vi "Login.vi"(7 "Database":refnum<queue>, 8 "error in (no error)":errorcluster, 11 "System Config":T1 {"Config Settings"."Simulated Sensor Injection" scale=0.0..100.0}) -> (0 "error out":errorcluster, 3 "Simulation Mode?":bool)   [LabVIEW 2026]
uses:
  Architecture/Message Queue/Message Cluster.ctl
  controls/UI/System Config.ctl
  controls/UI/Config Settings.ctl
  controls/UI/Analog Output.ctl
  controls/UI/Units Enum.ctl
  controls/UI/Signal Enum.ctl
  controls/UI/Login Refs.ctl
  controls/UI/UI List Type.ctl
  controls/Diagnostics/Error Payload.ctl
  controls/Diagnostics/Error Cluster.ctl
  controls/Messaging Payloads/Sensor InsertRequest.ctl
  controls/Messaging Payloads/Sensor CoreData Cluster.ctl
  controls/Messaging Payloads/Operator InsertRequest.ctl
  C:/Program Files (x86)/dotnet/shared/Microsoft.NETCore.App/8.0.22/System.Security.Cryptography.dll
  Program Files (x86)/dotnet/shared/Microsoft.NETCore.App/8.0.22/System.Security.Cryptography.dll
  Architecture/Message Queue/Enqueue Message (Single).vi
  Architecture/Message Queue/Message Queue.lvlib
  Settings/Settings.lvlib
panel:
  in  "Log Out":bool
  out "Message":string
  out "Status":bool
  in  "Tab Control":enum32{"Page 1", "Sensors", "Operators"}(tab)
  in  "OK Button":bool
  in  "Cancel Button":bool
  in  "Password":string
  in  "Output Signal":T4
  in  "Units":T5
  in  "Maximum":dbl
  in  "Minimum":dbl
  in  "Serial Number":string
  in  "Model Numbers":string(combo)
  in  "Submit":bool
  in  "Submit 2":bool
  in  "New Operator Name":string
  # "ADMINISTRATOR ACCESS"
  # "Enter you administrator password to continue."
  # "Administrator access is required to manage \n           sensors and operators."
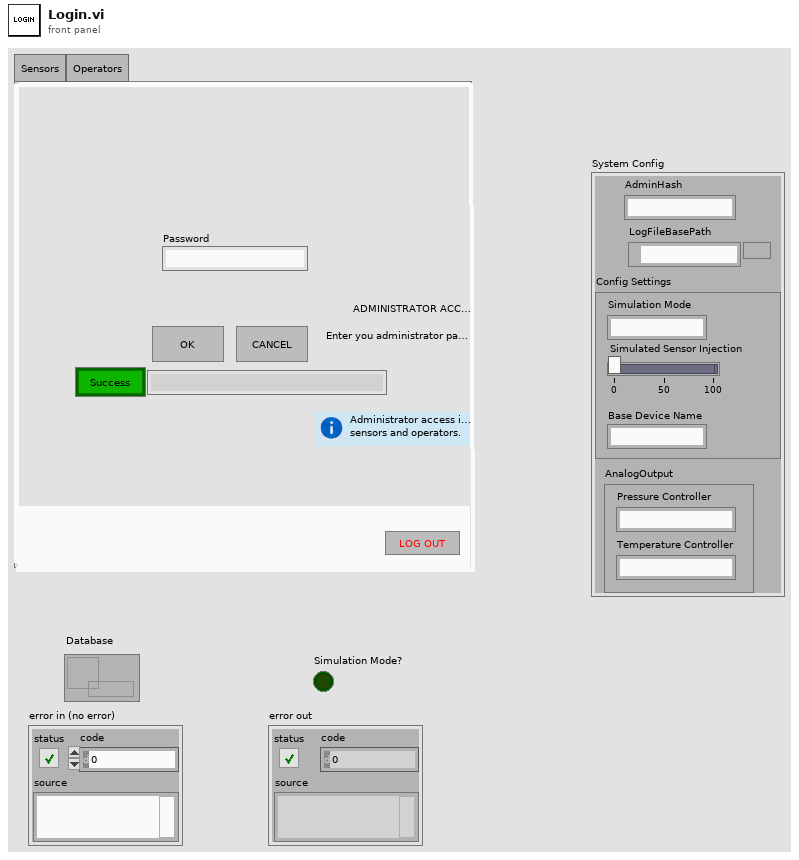
[diagram p1: front panel]
types:
  T1 = typedef "System Config.ctl" = cluster{"AdminHash":string, "LogFileBasePath ":path, "Config Settings":T2, "AnalogOutput":T3}
  T2 = typedef "Config Settings.ctl" = cluster{"Simulated Sensor Injection":dbl, "Base Device Name":string, "Simulation Mode":string}
  T3 = typedef "Settings.lvlib/Analog Output.ctl" = cluster{"Pressure Controller":string, "Temperature Controller":string}
  T4 = typedef "Signal Enum.ctl" = enum16{"4-20mA", "0-10V", "Thermocouple Type K"}
  T5 = typedef "Units Enum.ctl" = enum16{"PSI", "Deg C", "kPa", "GPM"}
  T6 = typedef "Login Refs.ctl" = cluster{"Serial Number Ref":refnum<vi>, "Submit Ref":refnum<vi>, "Clear Refnum ":refnum<vi>, "Logout Ref":refnum<vi>, "Message Ref":refnum<vi>, "Status Ref":refnum<vi>, "TabCtl Ref":refnum<vi>, "Submit Ref 2":refnum<vi>}
  T7 = enum8{"Enabled", "Disabled", "Disabled and Grayed Out"}
  T8 = typedef "UI List Type.ctl" = enum16{"Model Numbers", "Serial Numbers", "Operators", "Calibration Points", "Start Run Times"}
  T9 = typedef "Error Payload.ctl" = cluster{"Error Cluster":T10, "Message":string}
  T10 = typedef "Error Cluster.ctl" = errorcluster
  T11 = typedef "Sensor InsertRequest.ctl" = cluster{"Notifier":refnum<notifier>, "Sensor CoreData":T12}
  T12 = typedef "Settings.lvlib/Sensor CoreData Cluster.ctl" = cluster{"SensorID":i32, "SerialNumber":string, "ModelNumber":string, "Min":dbl, "Max":dbl, "Units":T5, "Output Signal":T4}
  T13 = typedef "Operator InsertRequest.ctl" = cluster{"Notifier":refnum<notifier>, "OperatorName":string, "BadgeNumber":string, "IsActive":i32}
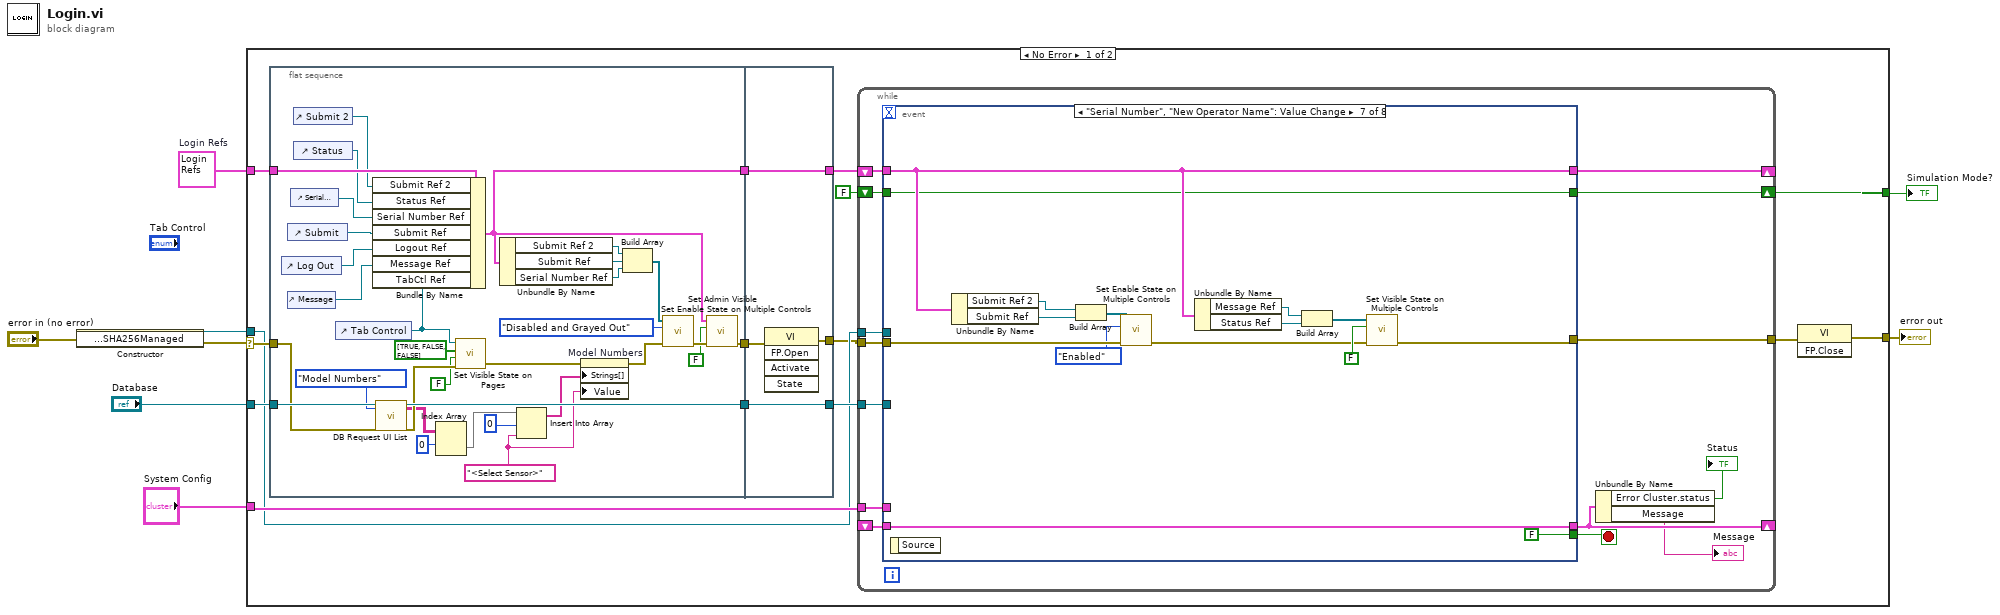
[diagram p0: block diagram]
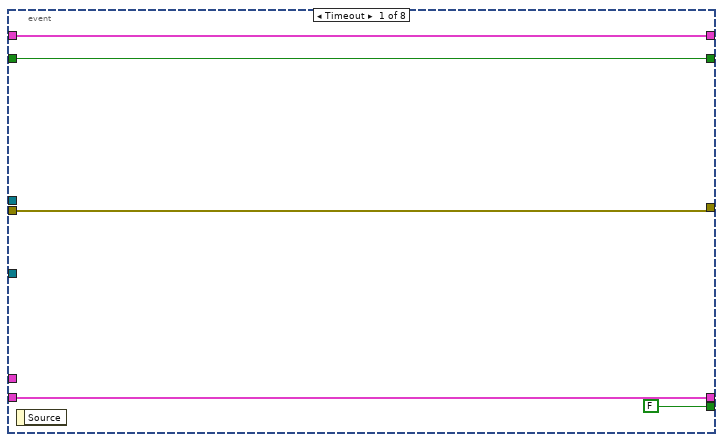
[diagram p2: hidden frame]
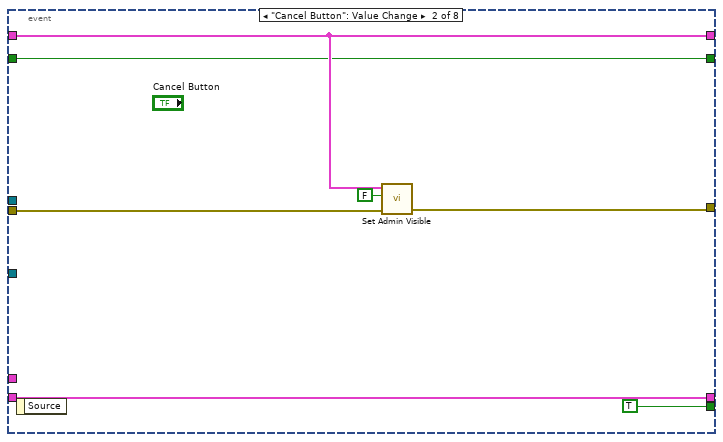
[diagram p3: hidden frame]
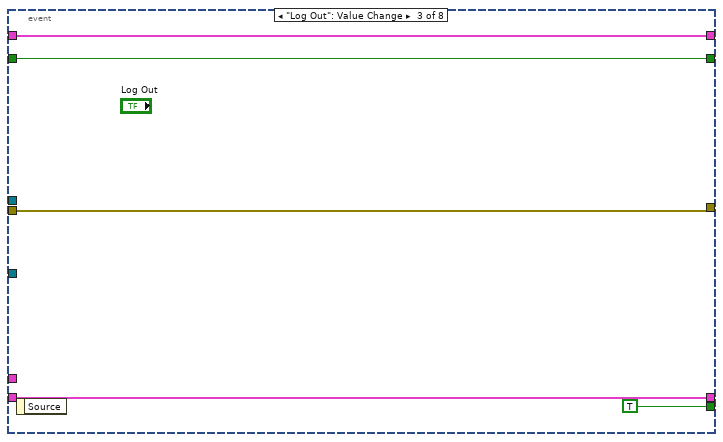
[diagram p4: hidden frame]
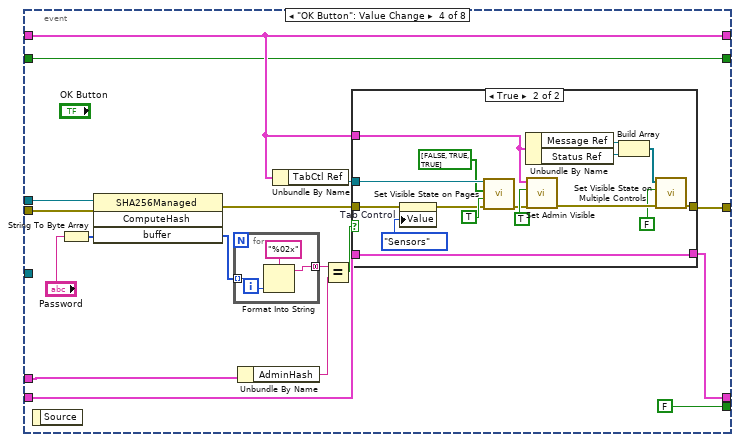
[diagram p5: hidden frame]
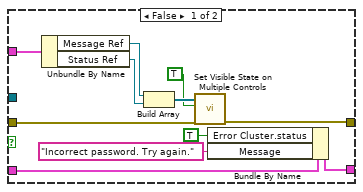
[diagram p6: hidden frame]
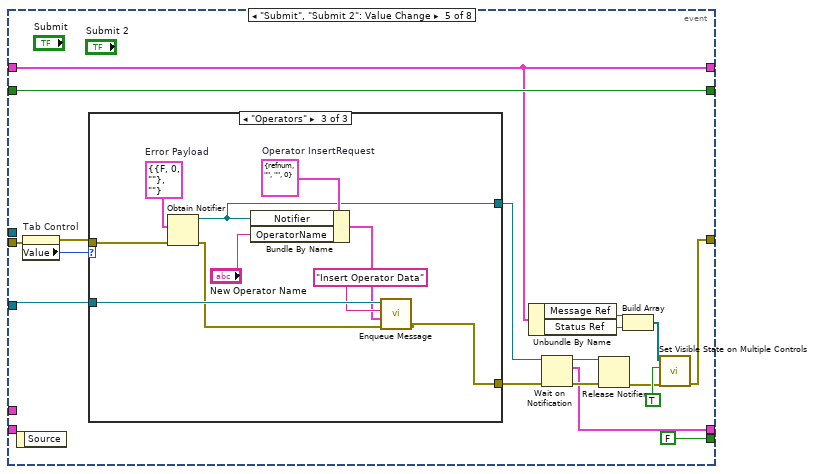
[diagram p7: hidden frame]
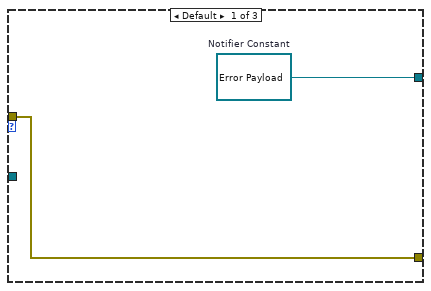
[diagram p8: hidden frame]
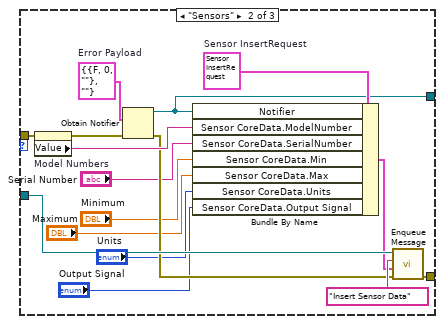
[diagram p9: hidden frame]
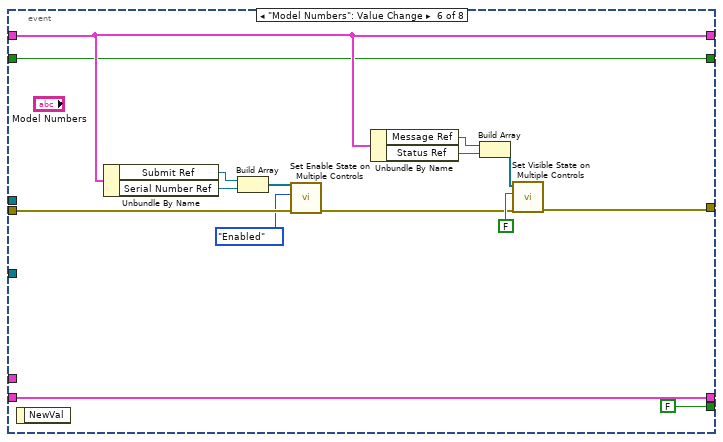
[diagram p10: hidden frame]
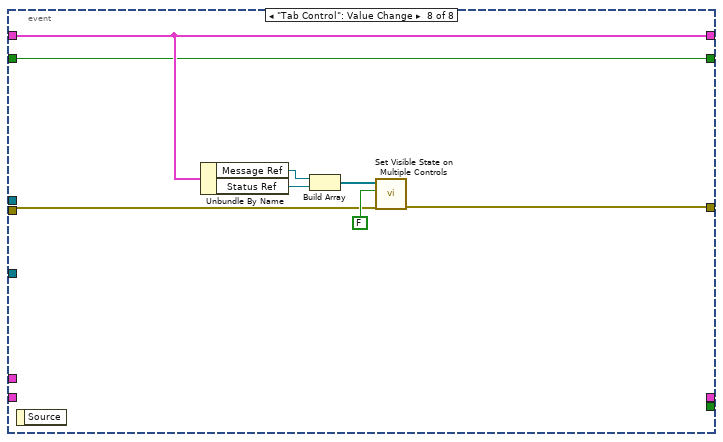
[diagram p11: hidden frame]
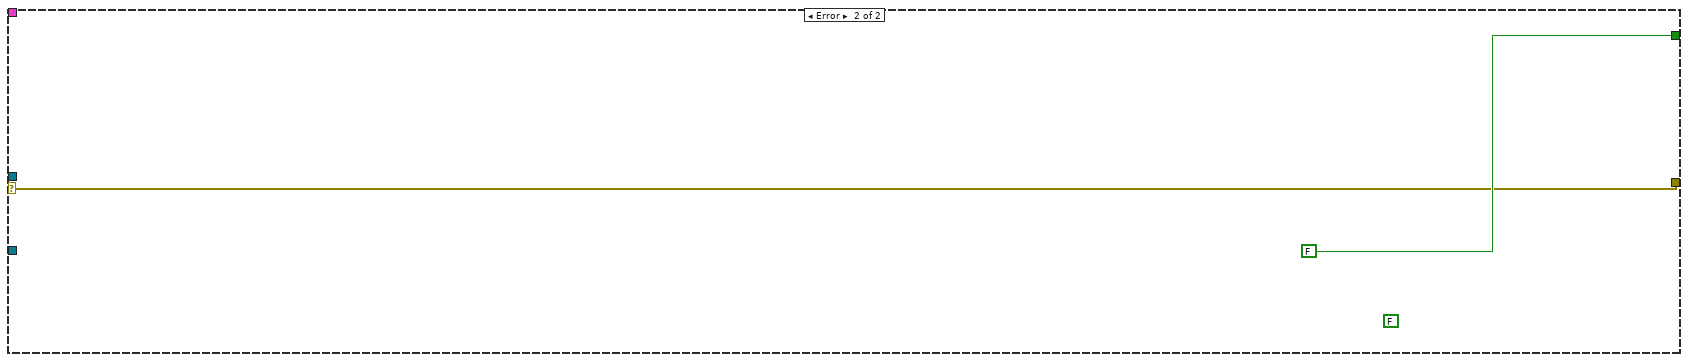
[diagram p12: hidden frame]
diagram:
  w3 = T6 {"Serial Number Ref"=refnum, "Submit Ref"=refnum, "Clear Refnum "=refnum, "Logout Ref"=refnum, "Message Ref"=refnum, "Status Ref"=refnum, "TabCtl Ref"=refnum, "Submit Ref 2"=refnum}  # Login Refs
  n1 = constructor class="SHA256Managed"(error in="error in (no error)") -> (reference out=w6:refnum<k39>, error out=w2:errorcluster)  [unwired: 2 in, 1 out]
  n2 = case shown="No Error" w2 {
    selector: w2 -> [w15 w222]
    tunnel: [w23 FALSE] -> w8
    tunnel: [w22 w222] -> w7
    tunnel: w6 -> [w14 _]
    tunnel: "Database" -> [w21 _]
    tunnel: w3 -> [w19 _]
    tunnel: "System Config" -> [w17 _]
    frame No Error {
      n3 = flat-sequence {
        tunnel: w21 -> [w55]
        tunnel: w19 -> [w50]
        tunnel: w15 -> [w32]
        tunnel: [w54] -> w13
        tunnel: [w39] -> w12
        tunnel: [w33] -> w11
        tunnel: [w58] -> w16
        tunnel: [w59] -> w20
        tunnel: w13 -> [w59]
        tunnel: w12 -> [w58]
        tunnel: w11 -> [w57]
        tunnel: [w56] -> w10
        frame #0 {
          w46 = "<Select Sensor>"
          n4 = control-ref of="Log Out"() -> (w51:refnum<vi>)
          n5 = control-ref of="Submit"() -> (w53:refnum<vi>)
          n6 = control-ref of="Message"() -> (w45:refnum<vi>)
          n7 = control-ref of="Serial Number"() -> (w52:refnum<vi>)
          n8 = control-ref of="Submit 2"() -> (w25:refnum<vi>)
          n9 = control-ref of="Status"() -> (w38:refnum<vi>)
          n10 = control-ref of="Tab Control"() -> (w26:refnum<vi>)
          n11 = Bundle By Name(cluster=w50, "Submit Ref 2"=w25, "Status Ref"=w38, "Serial Number Ref"=w52, "Submit Ref"=w53, "Logout Ref"=w51, "Message Ref"=w45, "TabCtl Ref"=w26) -> (w39:T6)
          n12 = call "DB Request UI List.vi"("Database in"=w55, "UI List Type"=UI_List_Type."Model Numbers", "error in (no error)"=w32) -> ("Database out"=w54:refnum<queue>, "Results"=w28:string[][], "error out"=w37:errorcluster)  [unwired: 14 in]
          n13 = Index Array(array=w28, index (row)=0 ("index")) -> (element=w27:string[])  [unwired: 1 in]
          n14 = call "Set Visible State on Pages.vi"("error in (no error)"=w37, "Tabs Visible?"=FALSE, "Pages Visible"=bool[] [TRUE, FALSE, FALSE] ("Visibles"), "TabControl in"=w26) -> ("error out"=w36:errorcluster)  [unwired: 7 in]
          n15 = Unbundle By Name(w39) -> ("Submit Ref 2"=w24:refnum<vi>, "Submit Ref"=w42:refnum<vi>, "Serial Number Ref"=w41:refnum<vi>)
          n16 = Insert Into Array(array=w27, index=0, new element=w46) -> (w47:string[])
          n17 = property on="Model Numbers" class="CmbBox"(error in=w36, "Strings[]"=w47, "Value"=w46) -> (error out=w48:errorcluster)  [unwired: 1 in, 1 out]
          n18 = Build Array(w24, w42, w41) -> (w43:refnum<vi>[])
          n19 = call "Set Enable State on Multiple Controls.vi"("Controls"=w43, "Disabled"=T7."Disabled and Grayed Out", "error in (no error)"=w48) -> ("error out"=w44:errorcluster)  [unwired: 7 in]
          n20 = call "Set Admin Visible .vi"("error in (no error)"=w44, "Visible"=FALSE, "Login Refs"=w39) -> ("error out"=w33:errorcluster)  [unwired: 8 in]
        }
        frame #1 {
          n21 = invoke class="VI" method="FP.Open"(error in=w57) -> (error out=w56:errorcluster)  [unwired: 4 in, 4 out]
        }
      }
      n22 = while {
        tunnel: w17 -> [w72]
        tunnel: w14 -> [w71]
        tunnel: w20 -> [w70]
        tunnel: w10 -> [w69]
        shift-right: [w65] -> _
        shift-left: _ -> [w67]
        shift-right: [w62] -> _
        shift-left: w16 -> [w63]
        tunnel: [w61] -> w18
        shift-right: [w73] -> w23
        shift-left: FALSE ("Simulation Mode") -> [w60]
        stop <- w68 stop-if-true
        n23 = event shown="[6] \"Serial Number\", \"New Operator Name\": Value Change" {
          selector: _ -> [_ _ _ _ _ _ _ _]
          dyn-events: _ -> [_ _ _ _ _ _ _ _]
          timeout: _ -> [_ _ _ _ _ _ _ _]
          tunnel: [w74 w79 w86 w91 w139 w186 w201 w214] -> w73
          tunnel: w72 -> [_ _ _ w98 _ _ _ _]
          tunnel: w71 -> [_ _ _ w106 _ _ _ _]
          tunnel: w69 -> [w77 w83 w89 w105 w147 w196 w211 w216]
          tunnel: w70 -> [_ _ _ _ w155 _ _ _]
          tunnel: [w77 w82 w89 w94 w141 w190 w202 w215] -> w61
          tunnel: [w76 w84 w88 w92 w149 w198 w213 _] -> w65
          tunnel: [FALSE ("status") TRUE TRUE FALSE FALSE ("status") FALSE ("status") FALSE ("status") _] -> w68
          tunnel: w67 -> [w76 w84 w88 w93 _ w198 w213 _]
          tunnel: w63 -> [w75 w81 w87 w95 w138 w189 w204 w217]
          tunnel: [w75 w81 w87 w95 w138 w189 w204 w217] -> w62
          tunnel: w60 -> [w74 w79 w86 w91 w139 w186 w201 w214]
          event Timeout {
            n24 = event-data() -> ()  [unwired: 1 in, 1 out]
          }
          event "Cancel Button": Value Change {
            n25 = event-data() -> ()  [unwired: 1 in, 1 out]
            n26 = call "Set Admin Visible .vi"("error in (no error)"=w83, "Visible"=FALSE, "Login Refs"=w81) -> ("error out"=w82:errorcluster)  [unwired: 8 in]
          }
          event "Log Out": Value Change {
            n27 = event-data() -> ()  [unwired: 1 in, 1 out]
          }
          event "OK Button": Value Change {
            n28 = event-data() -> ()  [unwired: 1 in, 1 out]
            n29 = String To Byte Array(string="Password") -> (unsigned byte array=w104:u8[])
            n30 = invoke class="SHA256Managed" method="ComputeHash"(reference=w106, error in=w105, "buffer"=w104) -> (error out=w100:errorcluster, "buffer"=w103:u8[])  [unwired: 1 in, 2 out]
            n31 = for {
              tunnel: w103 -> [w136] mode=indexing
              tunnel: [w135] -> w102 mode=concatenating
              n32 = Format Into String(format string="%02x", w136) -> (resulting string=w135:string)  [unwired: 2 in, 1 out]
            }
            n33 = Unbundle By Name(w98) -> ("AdminHash"=w97:string)
            n34 = Unbundle By Name(w95) -> ("TabCtl Ref"=w96:refnum<vi>)
            n35 = Equal?(x=w102, y=w97) -> (x = y?=w101:bool)
            n36 = case shown="True" w101 {
              tunnel: w100 -> [w118 w121]
              tunnel: [w112 w123] -> w94
              tunnel: w96 -> [_ w134]
              tunnel: w95 -> [w117 w125]
              tunnel: w93 -> [w113 w122]
              tunnel: [w111 w122] -> w92
              frame False {
                n37 = Unbundle By Name(w117) -> ("Message Ref"=w116:refnum<vi>, "Status Ref"=w108:refnum<vi>)
                n38 = Build Array(w116, w108) -> (w115:refnum<vi>[])
                n39 = call "Set Visible State on Multiple Controls.vi"("error in (no error)"=w118, "Visible?"=TRUE, "Controls"=w115) -> ("error out"=w112:errorcluster)  [unwired: 8 in]
                n40 = Bundle By Name(cluster=w113, "Error Cluster.status"=TRUE, "Message"="Incorrect password. Try again.") -> (w111:T9)
              }
              frame True {
                n41 = property on="Tab Control" class="TabCtl (strict)"(error in=w121, "Value"=enum32{"Page 1", "Sensors", "Operators"}."Sensors" ("Tab Control")) -> (error out=w120:errorcluster)  [unwired: 1 in, 1 out]
                n42 = call "Set Visible State on Pages.vi"("error in (no error)"=w120, "Tabs Visible?"=TRUE, "Pages Visible"=bool[] [FALSE, TRUE, TRUE] ("Visibles"), "TabControl in"=w134) -> ("error out"=w124:errorcluster)  [unwired: 7 in]
                n43 = Unbundle By Name(w125) -> ("Message Ref"=w126:refnum<vi>, "Status Ref"=w129:refnum<vi>)
                n44 = call "Set Admin Visible .vi"("error in (no error)"=w124, "Visible"=TRUE, "Login Refs"=w125) -> ("error out"=w130:errorcluster)  [unwired: 8 in]
                n45 = Build Array(w126, w129) -> (w128:refnum<vi>[])
                n46 = call "Set Visible State on Multiple Controls.vi"("error in (no error)"=w130, "Visible?"=FALSE, "Controls"=w128) -> ("error out"=w123:errorcluster)  [unwired: 8 in]
              }
            }
          }
          event "Submit", "Submit 2": Value Change {
            n47 = event-data() -> ()  [unwired: 1 in, 1 out]
            n48 = property on="Tab Control" class="TabCtl (strict)"(error in=w147) -> (error out=w146:errorcluster, "Value"=w148:enum32{"Page 1", "Sensors", "Operators"})  [unwired: 1 in, 1 out]
            n49 = case shown="\"Operators\"" w148 {
              tunnel: w155 -> [_ w173 w183]
              tunnel: w146 -> [w157 w169 w175]
              tunnel: [w157 w167 w174] -> w153
              tunnel: [w156 w160 w177] -> w151
              frame Default {
                w156 = refnum<notifier> refnum  # Notifier Constant
              }
              frame "Sensors" {
                w164 = T9 {"Error Cluster"={"status"=FALSE, "code"=0, "source"=""}, "Message"=""}  # Error Payload
                w171 = T11 {"Notifier"=refnum, "Sensor CoreData"={"SensorID"=0, "SerialNumber"="", "ModelNumber"="", "Min"=0.0, "Max"=0.0, "Units"=enum."PSI", "Output Signal"=enum."4-20mA"}}  # Sensor InsertRequest
                n50 = property on="Model Numbers" class="CmbBox"(error in=w169) -> (error out=w168:errorcluster, "Value"=w166:string)  [unwired: 1 in, 1 out]
                n51 = Obtain Notifier(notification data type=w164, error in (no error)=w168) -> (notifier out=w160:refnum<notifier>, error out=w165:errorcluster)  [unwired: 2 in, 1 out]
                n52 = Bundle By Name(cluster=w171, "Notifier"=w160, "Sensor CoreData.ModelNumber"=w166, "Sensor CoreData.SerialNumber"="Serial Number", "Sensor CoreData.Min"="Minimum", "Sensor CoreData.Max"="Maximum", "Sensor CoreData.Units"="Units", "Sensor CoreData.Output Signal"="Output Signal") -> (w170:T11)
                n53 = call-poly "Enqueue Message.vi"("error in (no error)"=w165, "Message Data"=w170, "Message"="Insert Sensor Data", "Message Queue"=w173) -> ("error out"=w167:errorcluster)  [unwired: 6 in, 1 out]
              }
              frame "Operators" {
                w178 = T9 {"Error Cluster"={"status"=FALSE, "code"=0, "source"=""}, "Message"=""}  # Error Payload
                w181 = T13 {"Notifier"=refnum, "OperatorName"="", "BadgeNumber"="", "IsActive"=0}  # Operator InsertRequest
                n54 = Obtain Notifier(notification data type=w178, error in (no error)=w175) -> (notifier out=w177:refnum<notifier>, error out=w179:errorcluster)  [unwired: 2 in, 1 out]
                n55 = Bundle By Name(cluster=w181, "Notifier"=w177, "OperatorName"="New Operator Name") -> (w180:T13)
                n56 = call-poly "Enqueue Message.vi"("error in (no error)"=w179, "Message Data"=w180, "Message"="Insert Operator Data", "Message Queue"=w183) -> ("error out"=w174:errorcluster)  [unwired: 6 in, 1 out]
              }
            }
            n57 = Unbundle By Name(w138) -> ("Message Ref"=w140:refnum<vi>, "Status Ref"=w145:refnum<vi>)
            n58 = Wait on Notification(notifier=w151, error in (no error)=w153) -> (notifier out=w152:refnum<notifier>, notification=w149:T9, error out=w154:errorcluster)  [unwired: 2 in, 1 out]
            n59 = Release Notifier(notifier=w152, error in (no error)=w154) -> (error out=w142:errorcluster)  [unwired: 1 in, 2 out]
            n60 = Build Array(w140, w145) -> (w144:refnum<vi>[])
            n61 = call "Set Visible State on Multiple Controls.vi"("error in (no error)"=w142, "Visible?"=TRUE, "Controls"=w144) -> ("error out"=w141:errorcluster)  [unwired: 8 in]
          }
          event "Model Numbers": Value Change {
            n62 = event-data() -> ()  [unwired: 1 in, 1 out]
            n63 = Unbundle By Name(w189) -> ("Submit Ref"=w185:refnum<vi>, "Serial Number Ref"=w195:refnum<vi>)
            n64 = Build Array(w185, w195) -> (w194:refnum<vi>[])
            n65 = call "Set Enable State on Multiple Controls.vi"("Controls"=w194, "Disabled"=T7."Enabled", "error in (no error)"=w196) -> ("error out"=w191:errorcluster)  [unwired: 7 in]
            n66 = Unbundle By Name(w189) -> ("Message Ref"=w187:refnum<vi>, "Status Ref"=w188:refnum<vi>)
            n67 = Build Array(w187, w188) -> (w193:refnum<vi>[])
            n68 = call "Set Visible State on Multiple Controls.vi"("error in (no error)"=w191, "Visible?"=FALSE, "Controls"=w193) -> ("error out"=w190:errorcluster)  [unwired: 8 in]
          }
          event "Serial Number", "New Operator Name": Value Change {
            n69 = event-data() -> ()  [unwired: 1 in, 1 out]
            n70 = Unbundle By Name(w204) -> ("Submit Ref 2"=w199:refnum<vi>, "Submit Ref"=w209:refnum<vi>)
            n71 = Build Array(w199, w209) -> (w210:refnum<vi>[])
            n72 = call "Set Enable State on Multiple Controls.vi"("Controls"=w210, "Disabled"=T7."Enabled", "error in (no error)"=w211) -> ("error out"=w203:errorcluster)  [unwired: 7 in]
            n73 = Unbundle By Name(w204) -> ("Message Ref"=w205:refnum<vi>, "Status Ref"=w206:refnum<vi>)
            n74 = Build Array(w205, w206) -> (w208:refnum<vi>[])
            n75 = call "Set Visible State on Multiple Controls.vi"("error in (no error)"=w203, "Visible?"=FALSE, "Controls"=w208) -> ("error out"=w202:errorcluster)  [unwired: 8 in]
          }
          event "Tab Control": Value Change {
            n76 = event-data() -> ()  [unwired: 1 in, 1 out]
            n77 = Unbundle By Name(w217) -> ("Message Ref"=w218:refnum<vi>, "Status Ref"=w219:refnum<vi>)
            n78 = Build Array(w218, w219) -> (w221:refnum<vi>[])
            n79 = call "Set Visible State on Multiple Controls.vi"("error in (no error)"=w216, "Visible?"=FALSE, "Controls"=w221) -> ("error out"=w215:errorcluster)  [unwired: 8 in]
          }
        }
        n80 = Unbundle By Name(w65) -> ("Error Cluster.status"=→"Status":bool, "Message"=→"Message":string)
      }
      n81 = invoke class="VI" method="FP.Close"(error in=w18) -> (error out=w22:errorcluster)  [unwired: 2 in, 2 out]
    }
    frame Error {
      (unwired) FALSE ("status")
    }
  }
  "error out" <- w7
  "Simulation Mode?" <- w8
